vi "keccak.ip.ctrl.loop.vi"(11 "Reset":bool) -> ()   [LabVIEW 2021]
uses:
  <vilib>/Platform/TimedLoop/XDataNode/timing_clust.ctl
  <vilib>/Platform/TimedLoop/XDataNode/nitl_modes.ctl
  <vilib>/Platform/TimedLoop/XDataNode/wakeup.ctl
  Users/johns/OneDrive/Documents/LabVIEW Data/Untitled Project 2/CLIP/keccak.variables.ctl
  Users/johns/OneDrive/Documents/LabVIEW Data/Untitled Project 2/CLIP/keccak.states.ctl
  <vilib>/rvi/Emulation/niFpgaSctlEmulationGetInTimedLoop.vi
  <vilib>/rvi/Emulation/niFpgaEmulationReportErrorSimple.vi
  <vilib>/rvi/Emulation/niFpgaGetClockAttributes.vi
  <vilib>/rvi/Emulation/niFpgaCriticalErrorInLSC.vi
  <vilib>/platform/TimedLoop/XDataNode/XDataNode.xnode
  <vilib>/Platform/TimedLoop/XDataNode/XDNodeRunTimeDep.lvlib
panel:
  in  "HT_DATA.Valid":bool
  in  "HT_DATA.Data":u64
  in  "HT_PARMS.Valid":bool
  in  "HT_PARMS.Data":u64
  in  "TH_RESULTS.Ready":bool
  out "Read.HT_DATA":bool
  out "Read.HT_PARMS":bool
  out "TH_RESULTS.Valid":bool
  out "TH_RESULTS.Data":u64
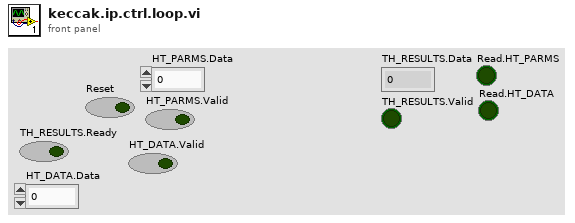
[diagram p1: front panel]
types:
  T1 = typedef "XDNodeRunTimeDep.lvlib/timing_clust.ctl" = cluster{"Expected End [f-1]":u64, "Actual End [f-1]":u64, "Finished Late? [f-1]":bool, "Expected End [i-1]":u64, "Actual End [i-1]":u64, "Finished Late? [i-1]":bool, "Expected Start [i]":u64, "Actual Start [i]":u64, "Expected Start [f]":u64, "Actual Start [f]":u64, "Source Name":string, "Structure Name":string, "Period":i64, "Deadline":i64, "Offset":i64, "Start":i64, "Priority":i32, "Timeout":i32, "Mode":T2, "Wakeup Reason":T3, "Error":errorcluster, "Source Type":string, "Secondary Source Type":string, "Global End Time":u64, "Global Start Time":u64, "Frame Duration":u64, "Iteration Duration":u64, "Assigned CPU":i32, "I/O Scan Engine Mode":u32}
  T2 = typedef "XDNodeRunTimeDep.lvlib/nitl_modes.ctl" = enum32{"No Change", "Process missed periods, maintain original phase", "Discard missed periods, maintain original phase", "Process missed periods, ignore original phase", "Discard missed periods, ignore original phase"}
  T3 = typedef "XDNodeRunTimeDep.lvlib/wakeup.ctl" = enum32{"Normal", "Aborted", "Asynchronous wakeup", "Timing source error", "Timed loop error", "Timeout"}
  T4 = typedef "keccak.variables.ctl" = cluster{"hash.input_size":u16, "hash.bits":u16, "state.next":T5, "state.after_next":T5, "read.i":u16, "read.block_i":u16, "hash.block_words":u16, "hash.block_size":u16, "keccak.i":u16, "state[25]":u64[], "HT_PARMS.Valid":bool, "HT_PARMS.Data":u64, "Read.HT_PARMS":bool, "HT_DATA.Valid":bool, "HT_DATA.Data":u64, "Read.HT_DATA":bool, "TH_RESULTS.Valid":bool, "TH_RESULTS.Data":u64, "TH_RESULTS.Ready":bool}
  T5 = typedef "keccak.states.ctl" = enum8{"Wait.for.Start", "Read.Blocks", "Read.Remainder", "Keccak", "Send.Result"}
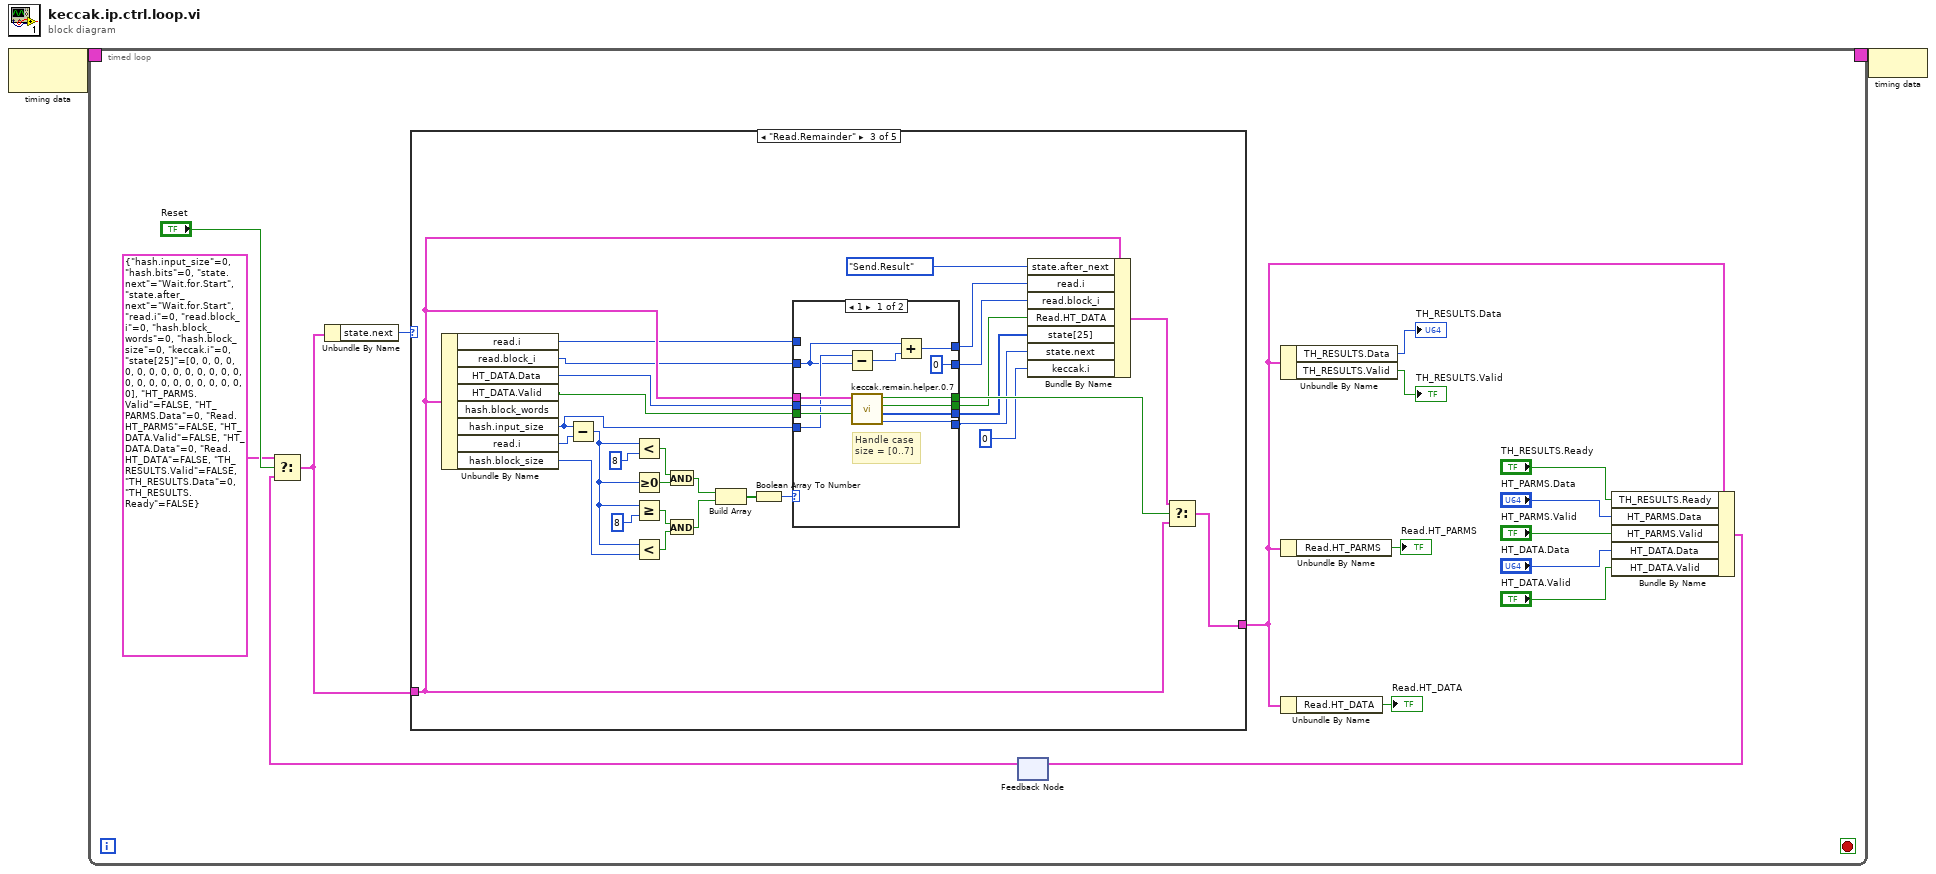
[diagram p0: block diagram]
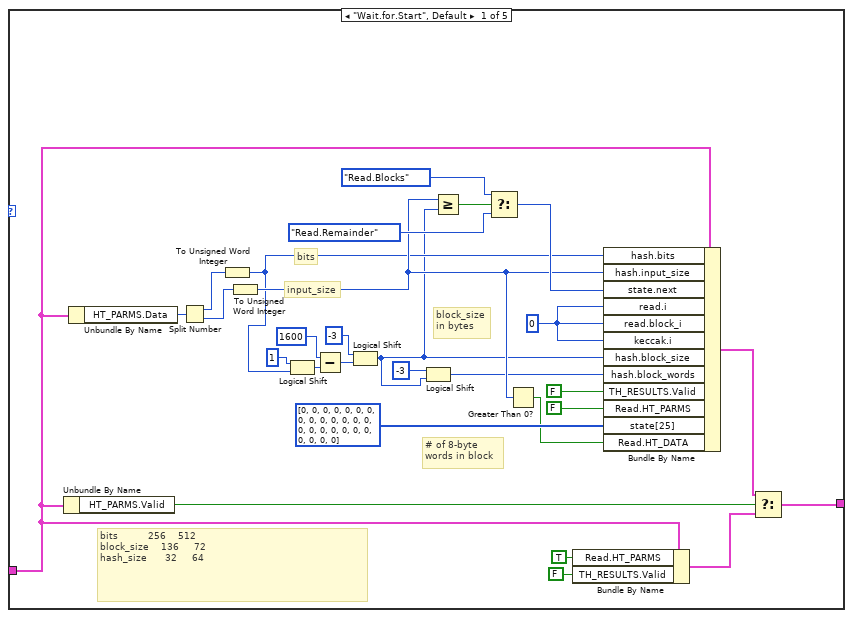
[diagram p2: hidden frame]
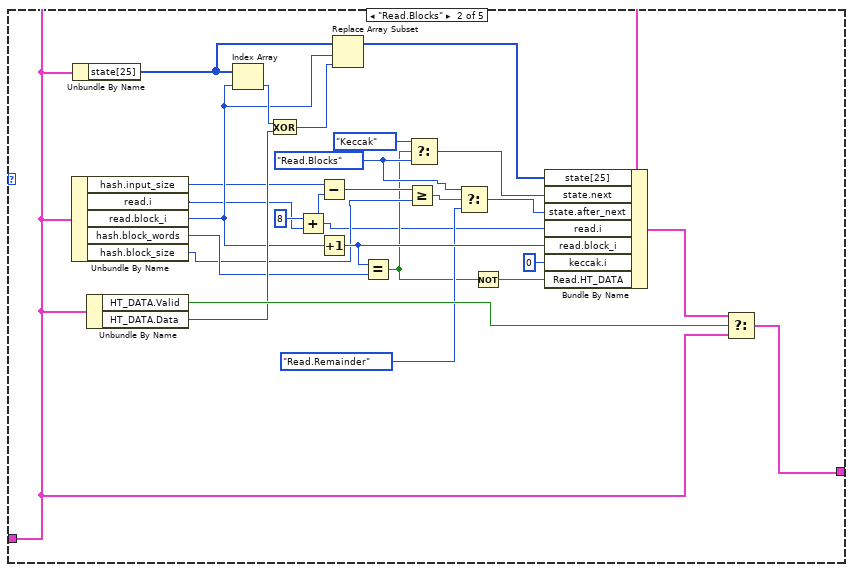
[diagram p3: hidden frame]
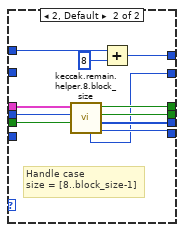
[diagram p4: hidden frame]
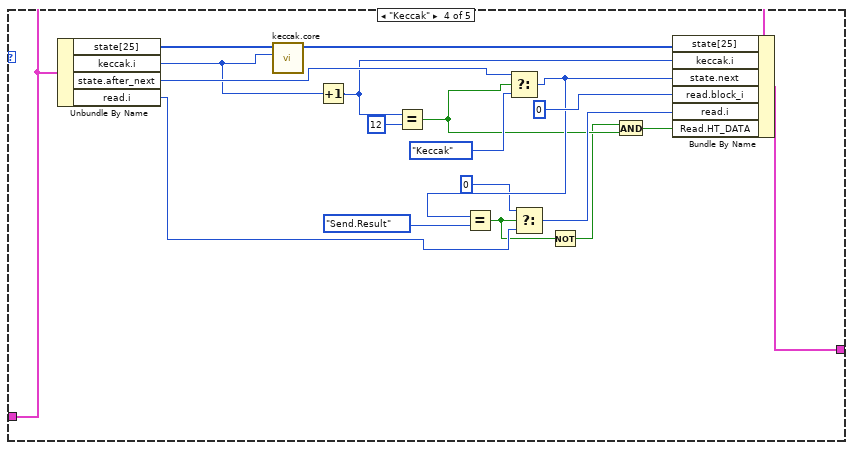
[diagram p5: hidden frame]
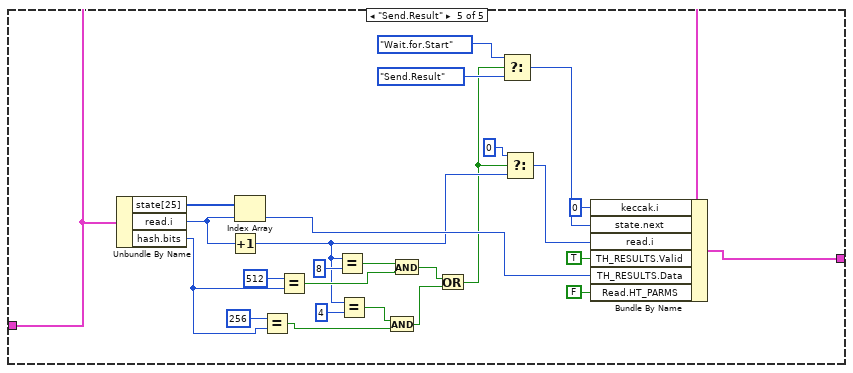
[diagram p6: hidden frame]
diagram:
  n1 = node-c288() -> (w2:T1)  [unwired: 1 in]
  n2 = timed-loop {
    timing: w2 -> [_]
    timing-out: [_] -> w1
    stop <- _ stop-if-true
    n3 = feedback #1() -> (w13:T4)  [unwired: 1 in]
    n4 = Select(t=T4 {"hash.input_size"=0, "hash.bits"=0, "state.next"=enum."Wait.for.Start", "state.after_next"=enum."Wait.for.Start", "read.i"=0, "read.block_i"=0, "hash.block_words"=0, "hash.block_size"=0, "keccak.i"=0, "state[25]"=[0, 0, 0, 0, 0, 0, 0, 0, 0, 0, 0, 0, 0, 0, 0, 0, 0, 0, 0, 0, 0, 0, 0, 0, 0], "HT_PARMS.Valid"=FALSE, "HT_PARMS.Data"=0, "Read.HT_PARMS"=FALSE, "HT_DATA.Valid"=FALSE, "HT_DATA.Data"=0, "Read.HT_DATA"=FALSE, "TH_RESULTS.Valid"=FALSE, "TH_RESULTS.Data"=0, "TH_RESULTS.Ready"=FALSE} ("Variables"), s="Reset", f=w13) -> (s? t:f=w12:T4)
    n5 = Unbundle By Name(w12) -> ("state.next"=w18:T5)
    n6 = case shown="\"Read.Remainder\"" w18 {
      tunnel: [w43 w73 w100 w143 w171] -> w17
      tunnel: w12 -> [w38 w72 w96 w144 w170]
      frame "Wait.for.Start", Default {
        w28 = u16 0 ("read.i")
        # "# of 8-byte\nwords in block"
        # "block_size\nin bytes"
        # "bits"
        # "input_size"
        # "bits          256    512\nblock_size    136     72\nhash_size      32     64"
        n7 = Unbundle By Name(w38) -> ("HT_PARMS.Valid"=w42:bool)
        n8 = Unbundle By Name(w38) -> ("HT_PARMS.Data"=w47:u64)
        n9 = Split Number(x=w47) -> (hi(x)=w46:u32, lo(x)=w45:u32)
        n10 = To Unsigned Word Integer(number=w46) -> (unsigned 16bit integer=w20:u16)
        n11 = To Unsigned Word Integer(number=w45) -> (unsigned 16bit integer=w30:u16)
        n12 = Logical Shift(y=i16 1, x=w20) -> (x << y=w25:u16)
        n13 = Subtract(x=u16 1600, y=w25) -> (x-y=w24:u16)
        n14 = Logical Shift(y=i16 -3, x=w24) -> (x << y=w19:u16)
        n15 = Logical Shift(y=i16 -3, x=w19) -> (x << y=w21:u16)
        n16 = Greater Or Equal?(x=w30, y=w19) -> (x >= y?=w34:bool)
        n17 = Select(t=keccak.states."Read.Blocks" ("state.next"), s=w34, f=keccak.states."Read.Remainder" ("state.next")) -> (s? t:f=w32:T5)
        n18 = Greater Than 0?(x=w30) -> (x > 0?=w29:bool)
        n19 = Bundle By Name(cluster=w38, "Read.HT_PARMS"=TRUE, "TH_RESULTS.Valid"=FALSE) -> (w39:T4)
        n20 = Bundle By Name(cluster=w38, "hash.bits"=w20, "hash.input_size"=w30, "state.next"=w32, "read.i"=w28, "read.block_i"=w28, "keccak.i"=w28, "hash.block_size"=w19, "hash.block_words"=w21, "TH_RESULTS.Valid"=FALSE, "Read.HT_PARMS"=FALSE, "state[25]"=u64[] [0, 0, 0, 0, 0, 0, 0, 0, 0, 0, 0, 0, 0, 0, 0, 0, 0, 0, 0, 0, 0, 0, 0, 0, 0] ("state[24]"), "Read.HT_DATA"=w29) -> (w44:T4)
        n21 = Select(t=w44, s=w42, f=w39) -> (s? t:f=w43:T4)
      }
      frame "Read.Blocks" {
        w53 = keccak.states."Read.Blocks" ("state.next")
        n22 = Unbundle By Name(w72) -> ("hash.input_size"=w58:u16, "read.i"=w57:u16, "read.block_i"=w66:u16, "hash.block_words"=w62:u16, "hash.block_size"=w54:u16)
        n23 = Unbundle By Name(w72) -> ("state[25]"=w70:u64[])
        n24 = Unbundle By Name(w72) -> ("HT_DATA.Valid"=w71:bool, "HT_DATA.Data"=w67:u64)
        n25 = Index Array(array=w70, index=w66) -> (element=w69:u64)
        n26 = Exclusive Or(1:w67, 2:w69) -> (0:w68:u64)
        n27 = Add(x=u16 8, y=w57) -> (x+y=w48:u16)
        n28 = Subtract(x=w58, y=w48) -> (x-y=w55:u16)
        n29 = Increment(x=w66) -> (x+1=w63:u16)
        n30 = Replace Array Subset(array=w70, new element=w68, index=w66) -> (w59:u64[])
        n31 = Equal?(x=w63, y=w62) -> (x = y?=w50:bool)
        n32 = Greater Or Equal?(x=w55, y=w54) -> (x >= y?=w56:bool)
        n33 = Select(t=keccak.states."Keccak" ("state.next"), s=w50, f=w53) -> (s? t:f=w64:T5)
        n34 = Select(t=w53, s=w56, f=keccak.states."Read.Remainder" ("state.next")) -> (s? t:f=w60:T5)
        n35 = Not(x=w50) -> (.not. x?=w49:bool)
        n36 = Bundle By Name(cluster=w72, "state[25]"=w59, "state.next"=w64, "state.after_next"=w60, "read.i"=w48, "read.block_i"=w63, "keccak.i"=u16 0, "Read.HT_DATA"=w49) -> (w74:T4)
        n37 = Select(t=w74, s=w71, f=w72) -> (s? t:f=w73:T4)
      }
      frame "Read.Remainder" {
        n38 = Unbundle By Name(w96) -> ("read.i"=w80:u16, "read.block_i"=w81:u16, "HT_DATA.Data"=w95:u64, "HT_DATA.Valid"=w94:bool, "hash.input_size"=w79:u16, "read.i"=w103:u16, "hash.block_size"=w83:u16)  [unwired: 1 out]
        n39 = Subtract(x=w79, y=w103) -> (x-y=w84:u16)
        n40 = Less?(x=w84, y=u16 8) -> (x < y?=w92:bool)
        n41 = Greater Or Equal To 0?(x=w84) -> (x >= 0?=w93:bool)
        n42 = Greater Or Equal?(x=w84, y=u16 8) -> (x >= y?=w87:bool)
        n43 = Less?(x=w84, y=w83) -> (x < y?=w82:bool)
        n44 = And(x=w92, y=w93) -> (x .and. y?=w89:bool)
        n45 = And(x=w87, y=w82) -> (x .and. y?=w86:bool)
        n46 = Build Array(w89, w86) -> (w90:bool[])
        n47 = Boolean Array To Number(Boolean array=w90) -> (number=w88:u8)
        n48 = case shown="1" w88 {
          tunnel: [w115 w122] -> w99
          tunnel: [w114 w123] -> w98
          tunnel: [w113 w121] -> w97
          tunnel: w96 -> [w112 w126]
          tunnel: w95 -> [w111 w125]
          tunnel: w94 -> [w110 w124]
          tunnel: [w109 w117] -> w78
          tunnel: w81 -> [w106 _]
          tunnel: [u16 0 w116] -> w76
          tunnel: [w105 w119] -> w75
          tunnel: w80 -> [_ w118]
          tunnel: w79 -> [w107 _]
          frame 1 {
            # "Handle case\nsize = [0..7]"
            n49 = Subtract(x=w107, y=w106) -> (x-y=w104:u16)
            n50 = call "keccak.remain.helper.0.7.vi"("HT_DATA.Valid"=w110, "HT_DATA.Data"=w111, "Variables"=w112) -> ("state.next"=w109:T5, "state[25] out"=w113:u64[], "Continue?"=w114:bool, "Valid"=w115:bool)  [unwired: 5 in]
            n51 = Add(x=w106, y=w104) -> (x+y=w105:u16)
          }
          frame 2, Default {
            # "Handle case\nsize = [8..block_size-1]"
            n52 = call "keccak.remain.helper.8.block_size.vi"("HT_DATA.Valid"=w124, "HT_DATA.Data"=w125, "Variables"=w126) -> ("state.next"=w117:T5, "state[25] out"=w121:u64[], "Continue?"=w123:bool, "Valid"=w122:bool, "read.block_i"=w116:u16)  [unwired: 4 in]
            n53 = Add(x=w118, y=u16 8) -> (x+y=w119:u16)
          }
        }
        n54 = Bundle By Name(cluster=w96, "state.after_next"=keccak.states."Send.Result" ("state.next"), "read.i"=w75, "read.block_i"=w76, "Read.HT_DATA"=w98, "state[25]"=w97, "state.next"=w78, "keccak.i"=u16 0) -> (w101:T4)
        n55 = Select(t=w101, s=w99, f=w96) -> (s? t:f=w100:T4)
      }
      frame "Keccak" {
        n56 = Unbundle By Name(w144) -> ("state[25]"=w145:u64[], "keccak.i"=w137:u16, "state.after_next"=w139:T5, "read.i"=w134:u16)
        n57 = call "keccak.core.vi"("keccak.i"=w137, "state[25]"=w145) -> ("state[25].out"=w142:u64[])  [unwired: 9 in]
        n58 = Increment(x=w137) -> (x+1=w138:u16)
        n59 = Equal?(x=w138, y=u16 12) -> (x = y?=w130:bool)
        n60 = Select(t=w139, s=w130, f=keccak.states."Keccak" ("state.next")) -> (s? t:f=w133:T5)
        n61 = Equal?(x=w133, y=keccak.states."Send.Result" ("state.next")) -> (x = y?=w128:bool)
        n62 = Select(t=u16 0, s=w128, f=w134) -> (s? t:f=w135:u16)
        n63 = Not(x=w128) -> (.not. x?=w127:bool)
        n64 = And(x=w127, y=w130) -> (x .and. y?=w129:bool)
        n65 = Bundle By Name(cluster=w144, "state[25]"=w142, "keccak.i"=w138, "state.next"=w133, "read.block_i"=u16 0 ("read.i"), "read.i"=w135, "Read.HT_DATA"=w129) -> (w143:T4)
      }
      frame "Send.Result" {
        n66 = Unbundle By Name(w170) -> ("state[25]"=w169:u64[], "read.i"=w168:u16, "hash.bits"=w158:u16)
        n67 = Increment(x=w168) -> (x+1=w151:u16)
        n68 = Index Array(array=w169, index=w168) -> (element=w159:u64)
        n69 = Equal?(x=u16 256, y=w158) -> (x = y?=w155:bool)
        n70 = Equal?(x=u16 512, y=w158) -> (x = y?=w164:bool)
        n71 = Equal?(x=w151, y=u16 8) -> (x = y?=w165:bool)
        n72 = Equal?(x=w151, y=u16 4) -> (x = y?=w154:bool)
        n73 = And(x=w154, y=w155) -> (x .and. y?=w153:bool)
        n74 = And(x=w165, y=w164) -> (x .and. y?=w152:bool)
        n75 = Or(x=w152, y=w153) -> (x .or. y?=w149:bool)
        n76 = Select(t=keccak.states."Wait.for.Start" ("state.next"), s=w149, f=keccak.states."Send.Result" ("state.next")) -> (s? t:f=w161:T5)
        n77 = Select(t=u16 0, s=w149, f=w151) -> (s? t:f=w150:u16)
        n78 = Bundle By Name(cluster=w170, "keccak.i"=u16 0, "state.next"=w161, "read.i"=w150, "TH_RESULTS.Valid"=TRUE, "TH_RESULTS.Data"=w159, "Read.HT_PARMS"=FALSE) -> (w171:T4)
      }
    }
    n79 = Unbundle By Name(w17) -> ("TH_RESULTS.Data"=→"TH_RESULTS.Data":u64, "TH_RESULTS.Valid"=→"TH_RESULTS.Valid":bool)
    n80 = Unbundle By Name(w17) -> ("Read.HT_PARMS"=→"Read.HT_PARMS":bool)
    n81 = Unbundle By Name(w17) -> ("Read.HT_DATA"=→"Read.HT_DATA":bool)
    n82 = Bundle By Name(cluster=w17, "TH_RESULTS.Ready"="TH_RESULTS.Ready", "HT_PARMS.Data"="HT_PARMS.Data", "HT_PARMS.Valid"="HT_PARMS.Valid", "HT_DATA.Data"="HT_DATA.Data", "HT_DATA.Valid"="HT_DATA.Valid") -> (w16:T4)
    n83 = feedback-in #1(w16) -> ()
  }
  n84 = node-c288(w1) -> ()
